vi "Set Pane Origin.vi"(8 "error in (no error)":errorcluster, 9 "pane index (0)":i32, 10 "origin (0,0)":T1, 11 "VI (caller)":refnum<vi>) -> (0 "error out":errorcluster, 3 "VI dup":refnum<vi>)   [LabVIEW 2017]
uses:
  <vilib>/Utility/miscctls.llb/LVPointTypeDef.ctl
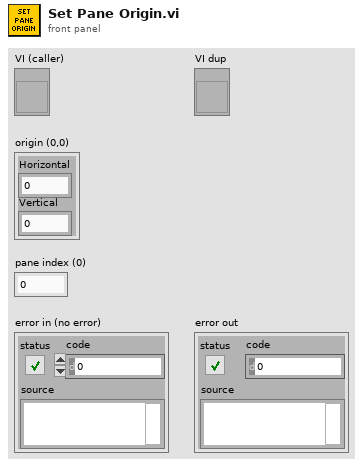
[diagram p1: front panel]
types:
  T1 = typedef "LVPointTypeDef.ctl" = cluster{"Horizontal":i16, "Vertical":i16}
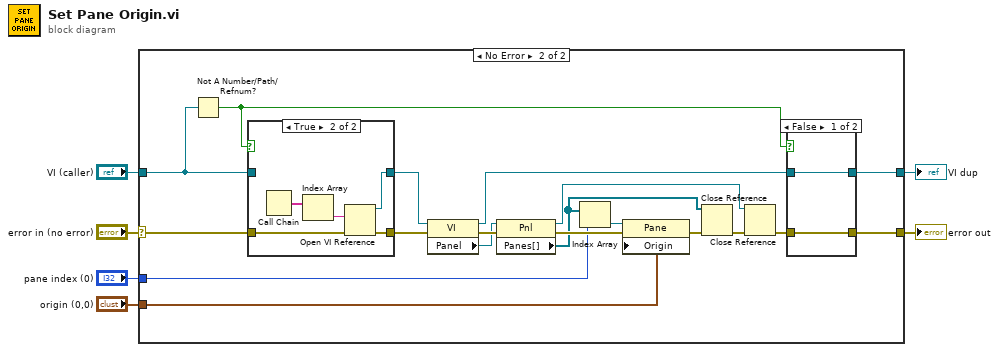
[diagram p0: block diagram]
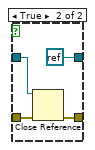
[diagram p3: hidden frame]
diagram:
  n1 = case shown="No Error" "error in (no error)" {
    selector: "error in (no error)" -> [w8 w16]
    tunnel: "origin (0,0)" -> [_ w21]
    tunnel: "pane index (0)" -> [_ w18]
    tunnel: "VI (caller)" -> [w7 w17]
    tunnel: [w7 w9] -> w3
    tunnel: [w8 w10] -> w1
    frame Error {
    }
    frame No Error {
      n2 = Not A Number/Path/Refnum?(number/path/refnum=w17) -> (NaN/Path/Refnum?=w13:bool)
      n3 = case shown="True" w13 {
        tunnel: w17 -> [w35 _]
        tunnel: w16 -> [w34 w38]
        tunnel: [w34 w37] -> w15
        tunnel: [w35 w36] -> w14
        frame False {
        }
        frame True {
          n4 = Call Chain() -> (call chain=w40:string[])
          n5 = Index Array(array=w40) -> (element=w39:string)  [unwired: 1 in]
          n6 = Open VI Reference(vi path=w39, error in (no error)=w38) -> (vi reference=w36:refnum<vi>, error out=w37:errorcluster)  [unwired: 4 in]
        }
      }
      n7 = property class="VI"(reference=w14, error in=w15) -> (reference out=w12:refnum<vi>, error out=w22:errorcluster, "Panel"=w19:refnum<vi>)
      n8 = property class="Pnl"(reference=w19, error in=w22) -> (reference out=w25:refnum<vi>, error out=w27:errorcluster, "Panes[]"=w26:refnum<vi>[])
      n9 = Index Array(array=w26, index=w18) -> (element=w20:refnum<vi>)
      n10 = property class="Pane"(reference=w20, error in=w27, "Origin"=w21) -> (error out=w23:errorcluster)  [unwired: 1 out]
      n11 = Close Reference(reference=w26, error in (no error)=w23) -> (error out=w24:errorcluster)
      n12 = Close Reference(reference=w25, error in (no error)=w24) -> (error out=w11:errorcluster)
      n13 = case shown="False" w13 {
        tunnel: w12 -> [w28 w33]
        tunnel: w11 -> [w29 w32]
        tunnel: [w29 w31] -> w10
        tunnel: [w28 refnum<k0> refnum] -> w9
        frame False {
        }
        frame True {
          n14 = Close Reference(reference=w33, error in (no error)=w32) -> (error out=w31:errorcluster)
        }
      }
    }
  }
  "VI dup" <- w3
  "error out" <- w1
